vi "All Running Vis.vi"(2 "Execution State (Run Top Level)":T1(ring)=enum."Run top level", 3 "Calling Vi path":path) -> (0 "Runnning Vi Names":string[](array[string]), 1 "Running Vi Paths":path[](array[path]))   [LabVIEW 2021, in "Utilities.lvlib"]
uses:
  Utilities.lvlib
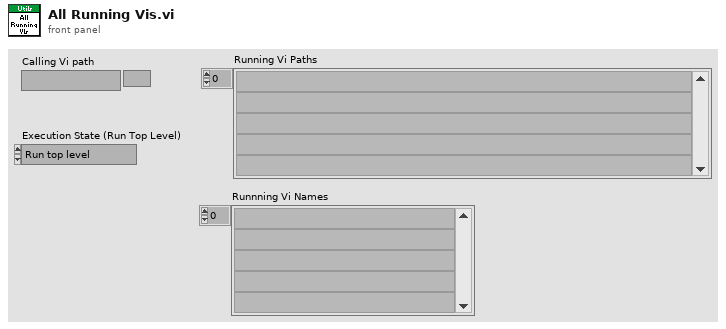
[diagram p1: front panel]
types:
  T1 = enum32{"Bad", "Idle", "Run top level", "Running"}
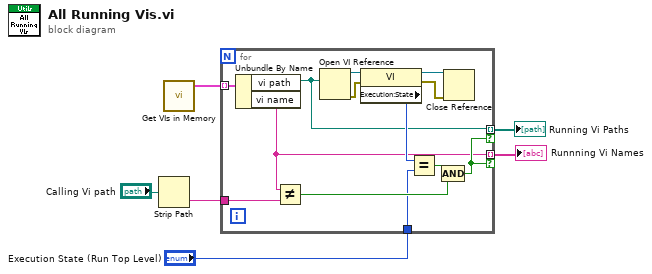
[diagram p0: block diagram]
diagram:
  n1 = Strip Path(path="Calling Vi path") -> (name=w4:string)  [unwired: 1 out]
  n2 = call "Get VIs in Memory.vi"() -> ("VIs in Memory"=w5:cluster{"vi name":string, "vi path":path}[])  [unwired: 4 in, 1 out]
  n3 = for {
    tunnel: w5 -> [w19] mode=indexing
    tunnel: w4 -> [w12]
    tunnel: "Execution State (Run Top Level)" -> [w10]
    tunnel: [w8] -> w2 mode=indexing if=w9
    tunnel: [w7] -> w1 mode=indexing if=w9
    n4 = Unbundle By Name(w19) -> ("vi path"=w8:path, "vi name"=w7:string)
    n5 = Not Equal?(x=w7, y=w12) -> (x != y?=w11:bool)
    n6 = Open VI Reference(vi path=w8) -> (vi reference=w18:refnum<vi>, error out=w15:errorcluster)  [unwired: 5 in]
    n7 = property class="VI"(reference=w18, error in=w15) -> (reference out=w17:refnum<vi>, error out=w16:errorcluster, "Execution:State"=w14:T1)
    n8 = Equal?(x=w14, y=w10) -> (x = y?=w13:bool)
    n9 = Compound Arithmetic op=AND(w13, w11) -> (w9:bool)
    n10 = Close Reference(reference=w17, error in (no error)=w16) -> ()  [unwired: 1 out]
  }
  "Runnning Vi Names" <- w1
  "Running Vi Paths" <- w2
